vi "ReadExternalInterfaces.vi"(8 "ErrorIn":errorcluster, 11 "DotNETCamIn":refnum<class "DotNETCam.lvclass">) -> (0 "ErrorOut":errorcluster, 2 "ExternalInterfaces":T1[](array[typedef]), 3 "DotNETCamOut":refnum<class "DotNETCam.lvclass">)   [LabVIEW 2021, in "DotNETCam.lvclass"]
uses:
  DotNETCam.lvclass
  .Externals/Library_TAF_Support/ClusterArrayConversion/BundledArray.ctl
  DotNETCam.lvclass/DotNETCam.ctl
  440278e9-1c04-4840-94c9-ed200201a6f0.vi
  440278e9-1c04-4840-94c9-ed200201a6f0.vi/e733eca7-9823-4359-8665-3b184f9a7377.vi
  <vilib>/Utility/Data Type/Get Cluster Information.vi
  <vilib>/Utility/Data Type/Get Type Information.vi
  .Externals/Library_TAF_Support/ClusterArrayConversion/ClusterArrayConversion.lvlib
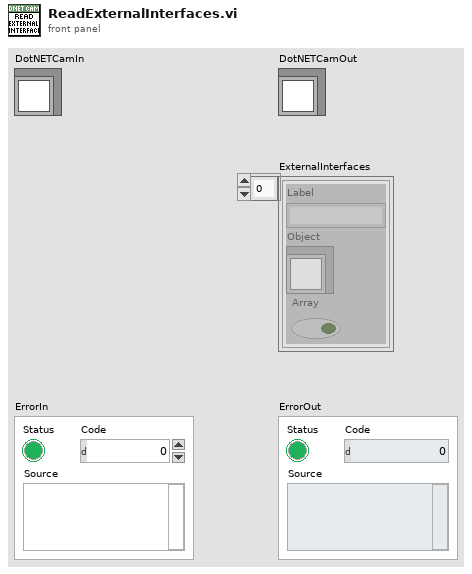
[diagram p1: front panel]
types:
  T1 = typedef "ClusterArrayConversion.lvlib/BundledArray.ctl" = cluster{"Label":string, "Object":refnum<class>, "Array":bool}
  T2 = cluster{"TAFObject":refnum<class "ITAFObject.lvclass">}
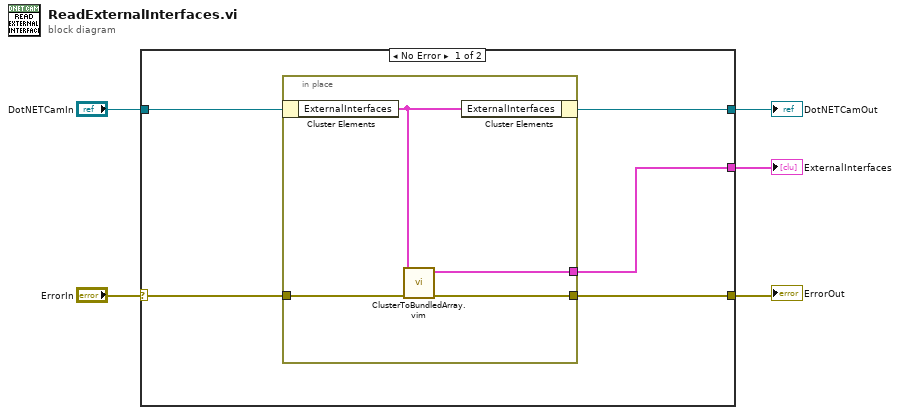
[diagram p0: block diagram]
diagram:
  n1 = case shown="No Error" "ErrorIn" {
    selector: "ErrorIn" -> [w10 w16]
    tunnel: [w9 w16] -> w4
    tunnel: [w7 w15] -> w2
    tunnel: "DotNETCamIn" -> [w8 w15]
    tunnel: [w6 _] -> w1
    frame No Error {
      n2 = in-place {
        in-place-border: w10 -> [w14]
        in-place-border: [w13] -> w9
        in-place-border: [w11] -> w6
        n3 = in-place-cluster #1(w8) -> ("ExternalInterfaces"=w12:T2)
        n4 = call "ClusterToBundledArray.vim"("ErrorIn"=w14, "Interfaces"=w12) -> ("ErrorOut"=w13:errorcluster, "BundeledLabels"=w11:T1[])  [unwired: 8 in]
        n5 = in-place-cluster #1("ExternalInterfaces"=w12) -> (w7:refnum<class "DotNETCam.lvclass">)
      }
    }
    frame Error {
    }
  }
  "ErrorOut" <- w4
  "DotNETCamOut" <- w2
  "ExternalInterfaces" <- w1
